vi "Close Report File.vi"(8 "error in (no error)":errorcluster, 11 "XML Report In":refnum<class "XML Report.lvclass">) -> (0 "error out":errorcluster, 2 "Report Path":path)   [LabVIEW 2020, in "XML Report.lvclass"]
uses:
  XML Report.lvclass
  Suite Result.ctl
  XML Report.lvclass/XML Report.ctl
  <vilib>/Utility/miscctls.llb/LVMapReplaceAction.ctl
  Core/Result/Status.ctl
  <vilib>/xml/Close Reference(Node).vi
  <vilib>/xml/NI_XML.lvlib
  Core/Result/Result.lvlib
  <vilib>/Platform/browser.llb/Open URL in Default Browser (path).vi
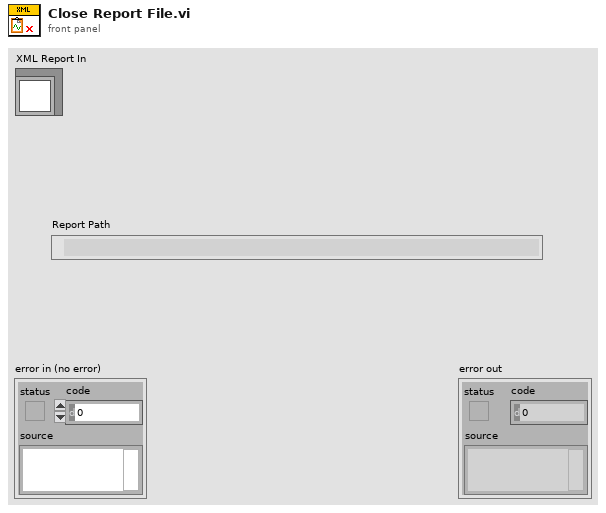
[diagram p1: front panel]
types:
  T1 = typedef "XML Report.lvclass/Suite Result.ctl" = cluster{"Name":string, "Tests":i32, "Failures":i32, "Execution Time":dbl}
  T2 = typedef "XML Report.lvclass/Case Result.ctl" = cluster{"Name":string, "Assertions":i32, "Classname":string, "Status":T3, "Time":dbl}
  T3 = typedef "Result.lvlib/Status.ctl" = enum16{"", "Passed", "Failed", "Error", "Skipped", "Setup Error", "Broken", "Teardown Error"}
  T4 = typedef "LVMapReplaceAction.ctl" = enum32{"Modify Entry only if found", "Add or Modify Entry", "Delete Entry"}
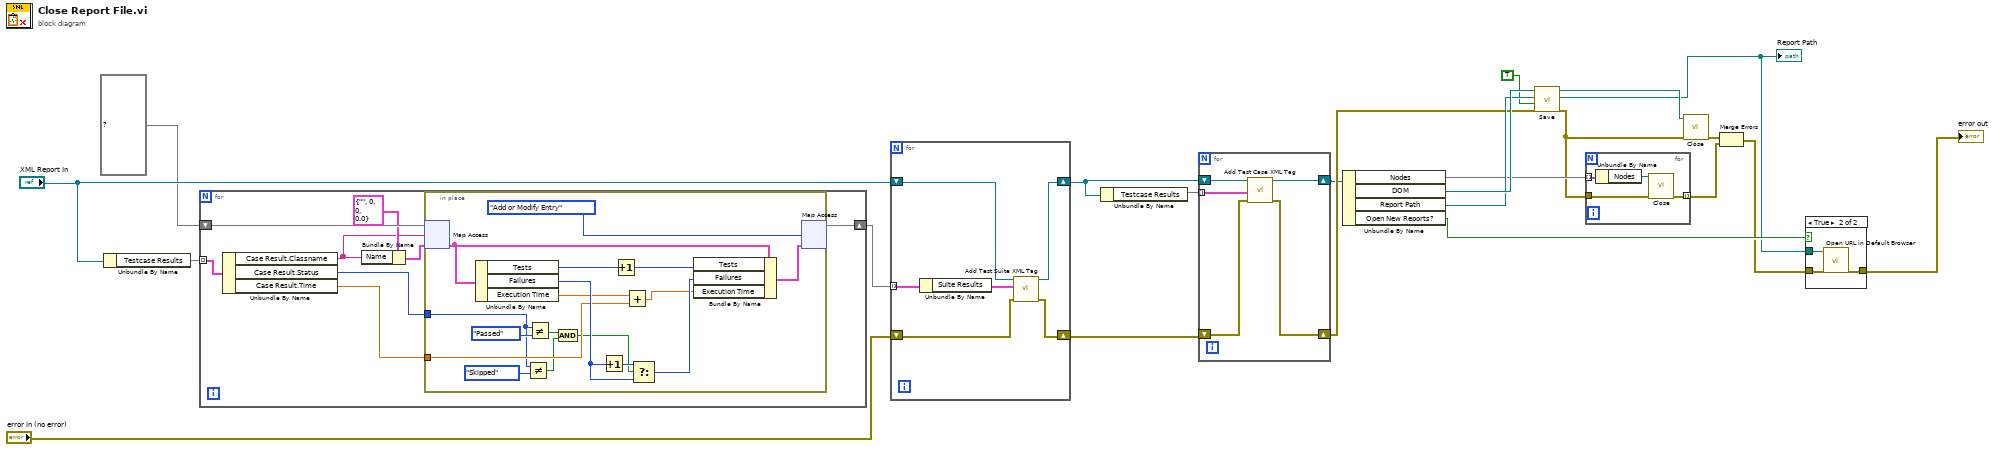
[diagram p0: block diagram]
diagram:
  n1 = Unbundle By Name("XML Report In") -> ("Testcase Results"=w8:map{string, T2})
  n2 = for {
    tunnel: w8 -> [w30] mode=indexing
    shift-right: [w29] -> w9
    shift-left: map{string, T1} {} ("map") -> [w28]
    n3 = Unbundle By Name(w30) -> ("Case Result.Classname"=w26:string, "Case Result.Status"=w24:T3, "Case Result.Time"=w23:dbl)
    n4 = Bundle By Name(cluster=T1 {"Name"="", "Tests"=0, "Failures"=0, "Execution Time"=0.0} ("value"), "Name"=w26) -> (w25:T1)
    n5 = in-place {
      in-place-border: w24 -> [w33]
      in-place-border: w23 -> [w37]
      n6 = in-place-map #1(w28, w26, w25) -> (w46:T1)  [unwired: 1 out]
      n7 = Unbundle By Name(w46) -> ("Tests"=w44:i32, "Failures"=w41:i32, "Execution Time"=w39:dbl)
      n8 = Not Equal?(x=w33, y=Status."Skipped" ("Status")) -> (x != y?=w32:bool)
      n9 = Not Equal?(x=w33, y=Status."Passed" ("Status")) -> (x != y?=w35:bool)
      n10 = And(x=w35, y=w32) -> (x .and. y?=w31:bool)
      n11 = Increment(x=w41) -> (x+1=w42:i32)
      n12 = Increment(x=w44) -> (x+1=w43:i32)
      n13 = Add(x=w39, y=w37) -> (x+y=w38:dbl)
      n14 = Select(t=w42, s=w31, f=w41) -> (s? t:f=w40:i32)
      n15 = Bundle By Name(cluster=w46, "Tests"=w43, "Failures"=w40, "Execution Time"=w38) -> (w45:T1)
      n16 = in-place-map #1(w45, LVMapReplaceAction."Add or Modify Entry" ("action")) -> (w29:map{string, T1})  [unwired: 2 out]
    }
  }
  n17 = for {
    shift-right: [w51] -> w6
    shift-left: "error in (no error)" -> [w52]
    shift-right: [w53] -> w5
    shift-left: "XML Report In" -> [w50]
    tunnel: w9 -> [w49] mode=indexing
    n18 = Unbundle By Name(w49) -> ("Suite Results"=w48:T1)
    n19 = call "Add Test Suite XML Tag.vi"("error in (no error)"=w52, "Suite Results"=w48, "Reports.lvlib:XML Report.lvclass"=w50) -> ("error out"=w51:errorcluster, "output cluster"=w53:refnum<class "XML Report.lvclass">)  [unwired: 7 in]
  }
  n20 = Unbundle By Name(w5) -> ("Testcase Results"=w7:map{string, T2})
  n21 = for {
    shift-right: [w55] -> w15
    shift-left: w6 -> [w56]
    shift-right: [w57] -> w14
    shift-left: w5 -> [w58]
    tunnel: w7 -> [w54] mode=indexing
    n22 = call "Add Test Case XML Tag.vi"("error in (no error)"=w56, "Test Case Result"=w54, "Reports.lvlib:XML Report.lvclass"=w58) -> ("error out"=w55:errorcluster, "output cluster"=w57:refnum<class "XML Report.lvclass">)  [unwired: 7 in]
  }
  n23 = Unbundle By Name(w14) -> ("Nodes"=w18:map{string, refnum<k20>}, "DOM"=w22:refnum<k20>, "Report Path"=w19:path, "Open New Reports?"=w4:bool)
  n24 = call <vilib>:"Save.vi"("error in (no error)"=w15, "overwrite file (True)"=TRUE, "XML file path"=w19, "DOM document in"=w22) -> ("error out"=w11:errorcluster, "XML file path out"=w1:path, "DOM document out"=w21:refnum<k20>)  [unwired: 5 in]
  "Report Path" <- w1
  n25 = for {
    tunnel: w18 -> [w62] mode=indexing
    tunnel: [w60] -> w17 mode=indexing
    tunnel: w11 -> [w59]
    n26 = Unbundle By Name(w62) -> ("Nodes"=w61:refnum<k20>)
    n27 = call-poly <vilib>:"Close.vi"("error in (no error)"=w59, "node"=w61) -> ("error out"=w60:errorcluster)  [unwired: 7 in]
  }
  n28 = call-poly <vilib>:"Close.vi"("error in (no error)"=w11, "node"=w21) -> ("error out"=w16:errorcluster)  [unwired: 7 in]
  n29 = Merge Errors(w16, w17) -> (w3:errorcluster)
  n30 = case shown="True" w4 {
    tunnel: w1 -> [_ w64]
    tunnel: w3 -> [w63 w66]
    tunnel: [w63 w65] -> w2
    frame False {
    }
    frame True {
      n31 = call-poly <vilib>:"Open URL in Default Browser.vi"("error in (no error)"=w66, "path"=w64) -> ("error out"=w65:errorcluster)  [unwired: 4 in, 1 out]
    }
  }
  "error out" <- w2
